vi "dbl to fr string small.vi"(7 "number":dbl) -> (8 "String":string)   [LabVIEW 2018]
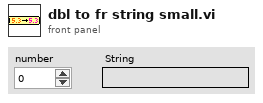
[diagram p1: front panel]
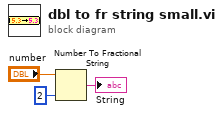
[diagram p0: block diagram]
diagram:
  n1 = Number To Fractional String(number="number", precision (6)=i16 2) -> (F-format string=→"String":string)  [unwired: 2 in]
